vi "TransformArrayTo16Bits.vi"(1 "Bytes In":u8[](array[numeric])) -> (0 "Byte Out":u16[](array[numeric]) format="%.0x")   [LabVIEW 2020, in "FirmataClient.lvlib"]
doc: "The Firmata protocol reserves the 8th bit of every packet for its own operation. So any data that must be transferred on the wire must be preprocessed. And on the receive side, these split packed must be reconstrusted. This is what this VI does.\n\nFor example a 8 bit data is split over 2 bytes, the first byte will contain the least significant 7bits, and the last 8th bit is placed in the other byte (i.e 0xFF becomes [ 0xEF, 0x01 ]). Then this VI reconstructs this as a 16byte number. It is up to the user to determine whether this 16byte representation is too much or not enough. For example, a char only needs 1byte, so the output of this VI is cast to that (See get firmware message parser)\n\nThe same logic can be applied for 16, 32,... bits data (0xFFAA becomes [ 0xEF, 0x01, 0x2A, 0x01 ])"
uses:
  FirmataClient.lvlib
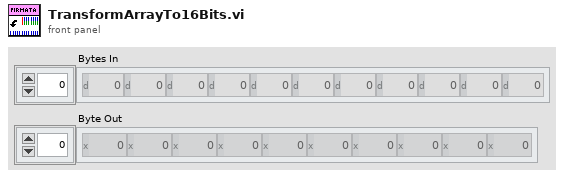
[diagram p1: front panel]
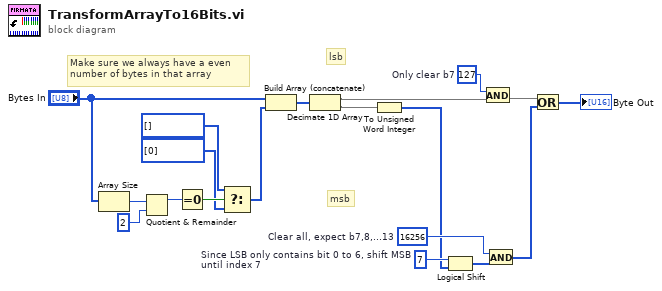
[diagram p0: block diagram]
diagram:
  w19 = u8 127  # Only clear b7
  w18 = u16 16256  # Clear all, expect b7,8,...13
  w16 = i16 7  # Since LSB only contains bit 0 to 6, shift MSB until index 7
  # "Make sure we always have a even \nnumber of bytes in that array"
  # "msb"
  # "lsb"
  n1 = Array Size(array="Bytes In") -> (size(s)=w14:i32)
  n2 = Quotient & Remainder(x=w14, y=2) -> (x-y*floor(x/y)=w10:i32)  [unwired: 1 out]
  n3 = Equal To 0?(x=w10) -> (x = 0?=w9:bool)
  n4 = Select(t=u8[] [] ("Bytes In"), s=w9, f=u8[] [0] ("Bytes In")) -> (s? t:f=w8:u8[])
  n5 = Build Array (concatenate)("Bytes In", w8) -> (w11:u8[])
  n6 = Decimate 1D Array(w11) -> (w15:u8[], w2:u8[])
  n7 = To Unsigned Word Integer(number=w2) -> (unsigned 16bit integer=w1:u16[])
  n8 = Logical Shift(y=w16, x=w1) -> (x << y=w17:u16[])
  n9 = And(x=w19, y=w15) -> (x .and. y?=w5:u8[])
  n10 = And(x=w18, y=w17) -> (x .and. y?=w4:u16[])
  n11 = Or(x=w5, y=w4) -> (x .or. y?=→"Byte Out":u16[])
